vi "ROI entry-Free hand same size.vi"(5 "Index of ROI end":i32, 7 "Index of ROI start":i32, 9 "Registered Line Coordinates":i32[](array[numeric]), 11 "Coordinates in":i32[](array[numeric])) -> (3 "Coordinates out":i32[](array[numeric]))   [LabVIEW 2020]
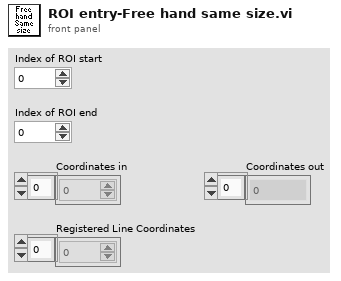
[diagram p1: front panel]
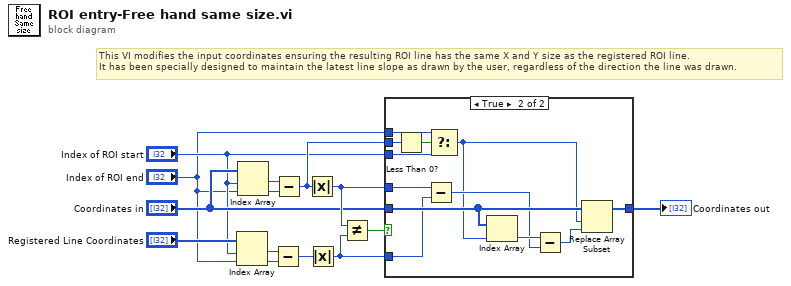
[diagram p0: block diagram]
diagram:
  # "This VI modifies the input coordinates ensuring the resulting ROI line has the same X and Y size as the registered ROI line.\nIt has been specially designed to maintain the latest line slope as drawn by the user, regardless of the direction the line was drawn."
  n1 = Index Array(array="Registered Line Coordinates", index #1="Index of ROI start", index #2="Index of ROI end") -> (element #1=w4:i32, element #2=w5:i32)
  n2 = Index Array(array="Coordinates in", index #1="Index of ROI start", index #2="Index of ROI end") -> (element #1=w8:i32, element #2=w7:i32)
  n3 = Subtract(x=w4, y=w5) -> (x-y=w11:i32)
  n4 = Subtract(x=w8, y=w7) -> (x-y=w14:i32)
  n5 = Absolute Value(x=w14) -> (abs(x)=w12:i32)
  n6 = Absolute Value(x=w11) -> (abs(x)=w13:i32)
  n7 = Not Equal?(x=w12, y=w13) -> (x != y?=w10:bool)
  n8 = case shown="True" w10 {
    tunnel: [w15 w22] -> w3
    tunnel: "Coordinates in" -> [w15 w27]
    tunnel: w12 -> [_ w26]
    tunnel: w13 -> [_ w25]
    tunnel: w14 -> [_ w20]
    tunnel: "Index of ROI end" -> [_ w17]
    tunnel: "Index of ROI start" -> [_ w16]
    frame False {
    }
    frame True {
      n9 = Less Than 0?(x=w20) -> (x < 0?=w19:bool)
      n10 = Subtract(x=w26, y=w25) -> (x-y=w21:i32)
      n11 = Select(t=w17, s=w19, f=w16) -> (s? t:f=w18:i32)
      n12 = Index Array(array=w27, index=w18) -> (element=w24:i32)
      n13 = Subtract(x=w24, y=w21) -> (x-y=w23:i32)
      n14 = Replace Array Subset(array=w27, new element=w23, index=w18) -> (w22:i32[])
    }
  }
  "Coordinates out" <- w3
